vi "Calculate-value-shape.vi"(4 "Center index X":i32, 5 "Temperature field":dbl[][](array[numeric]), 6 "Center index Y":i32, 7 "Characteristics":T2[](array[typedef]), 8 "error in":errorcluster, 10 "Temp. params. ref. in":refnum<data-value>, 11 "Config. params. ref. in":refnum<data-value>) -> (0 "error IO":errorcluster, 1 "Temperature characteristics":T1 {"Stand. dev. temperature" format="%#.1f"; "Min. temperature" format="%#.0f"; "Max. temperature" format="%#.0f"; "Average temperature" format="%#.0f"}, 2 "Temp. params. ref. in":refnum<data-value>, 3 "Config. params. ref.":refnum<data-value>)   [LabVIEW 2013, in "CameraVision.lvlib" / "CV-Temperature.lvclass"]
uses:
  CV-Temperature.lvclass
  Analysis/Characteristics-cluster.ctl
  Configuration/CV-Configuration.lvclass
  Temperature-characteristics.ctl
  Configuration/CV-Configuration.lvclass/CV-Configuration.ctl
  CV-Temperature.lvclass/CV-Temperature.ctl
  <vilib>/Analysis/coordinate.llb/2D Cartesian Coordinate Shift (Scalar).vi
  <vilib>/Analysis/coordinate.llb/2D Cartesian Coordinate Rotation (Scalar).vi
  Read Averaging shape.vi
  Read Major axis.vi
  Read Minor axis.vi
  Configuration/Read ROI width.vi
  Configuration/Read ROI height.vi
  <vilib>/Analysis/NI_AALPro.lvlib
  Analysis/CV-Analysis.lvclass
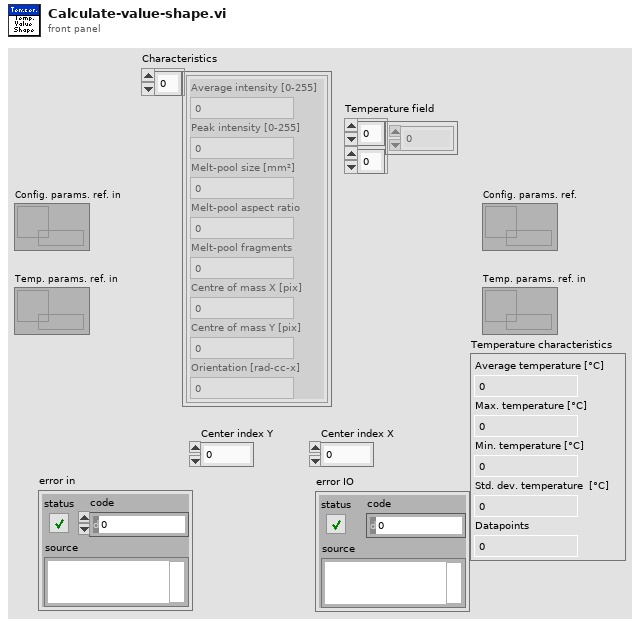
[diagram p1: front panel]
types:
  T1 = typedef "CameraVision.lvlib/CV-Temperature.lvclass/Temperature-characteristics.ctl" = cluster{"Average temperature ":dbl, "Max. temperature":dbl, "Min. temperature":dbl, "Stand. dev. temperature":dbl, "Datapoints":dbl}
  T2 = typedef "CameraVision.lvlib/CV-Analysis.lvclass/Characteristics-cluster.ctl" = cluster{"Average intensity":dbl, "Peak intensity":dbl, "Melt-pool size":dbl, "Melt-pool aspect ratio":dbl, "Melt-pool fragments":dbl, "Centre of mass X":dbl, "Centre of mass Y":dbl, "Orientation":dbl}
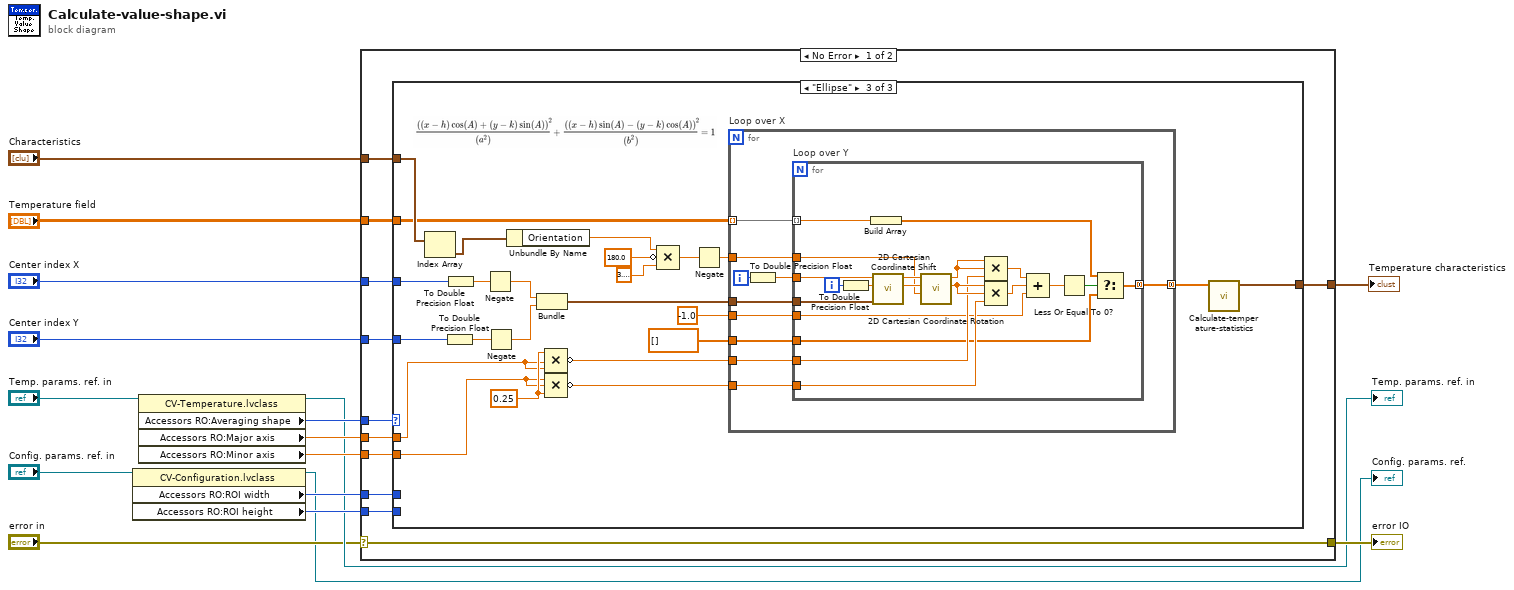
[diagram p0: block diagram]
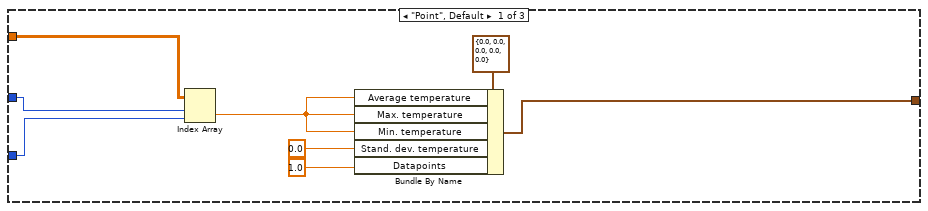
[diagram p2: hidden frame]
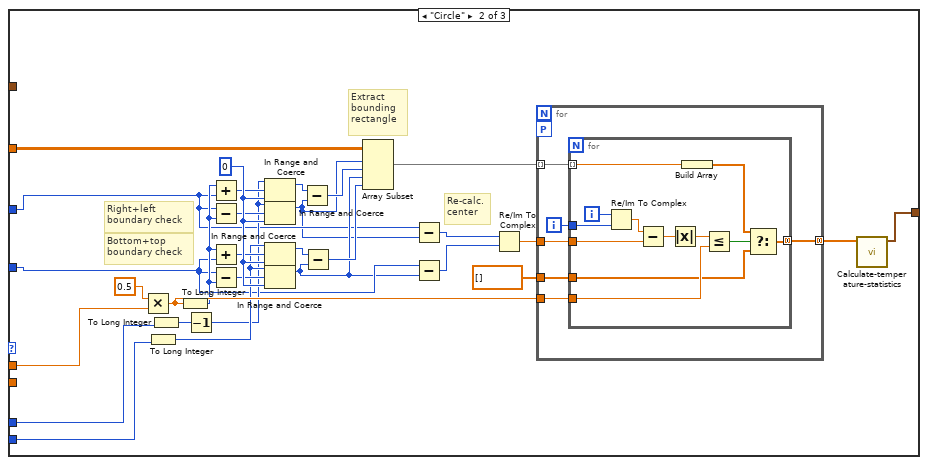
[diagram p3: hidden frame]
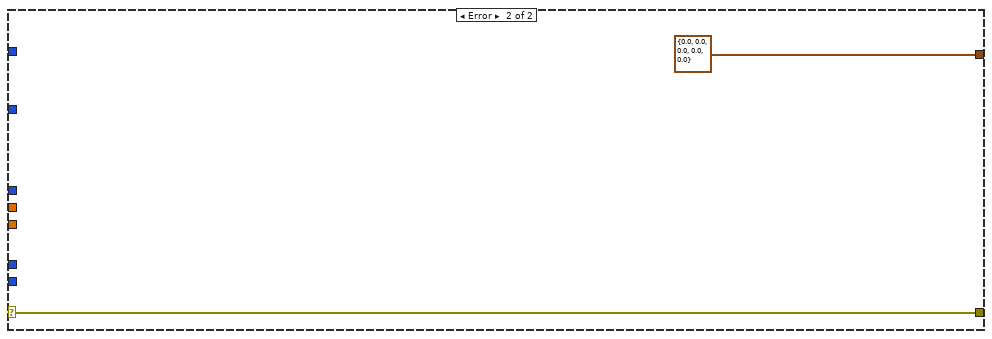
[diagram p4: hidden frame]
diagram:
  n1 = property class="CV-Configuration.lvclass"(reference="Config. params. ref. in") -> (reference out=→"Config. params. ref.":refnum<data-value>, "Accessors RO:ROI width"=w6:u32, "Accessors RO:ROI height"=w5:u32)  [unwired: 1 in, 1 out]
  n2 = property class="CV-Temperature.lvclass"(reference="Temp. params. ref. in") -> (reference out=→"Temp. params. ref. in":refnum<data-value>, "Accessors RO:Averaging shape"=w10:enum16{"Point", "Circle", "Ellipse"}, "Accessors RO:Major axis"=w9:dbl, "Accessors RO:Minor axis"=w8:dbl)  [unwired: 1 in, 1 out]
  n3 = case shown="No Error" "error in" {
    selector: "error in" -> [w23 w139]
    tunnel: [w27 T1 {"Average temperature "=0.0, "Max. temperature"=0.0, "Min. temperature"=0.0, "Stand. dev. temperature"=0.0, "Datapoints"=0.0} ("Temperature characteristics")] -> w2
    tunnel: "Center index Y" -> [w26 _]
    tunnel: "Center index X" -> [w25 _]
    tunnel: w10 -> [w24 _]
    tunnel: [w23 w139] -> w14
    tunnel: "Temperature field" -> [w22 _]
    tunnel: "Characteristics" -> [w21 _]
    tunnel: w9 -> [w20 _]
    tunnel: w8 -> [w19 _]
    tunnel: w6 -> [w18 _]
    tunnel: w5 -> [w17 _]
    frame No Error {
      n4 = case shown="\"Ellipse\"" w24 {
        tunnel: w25 -> [w35 w42 w106]
        tunnel: w26 -> [w34 w44 w105]
        tunnel: [w32 w62 w84] -> w27
        tunnel: w22 -> [w29 w40 w88]
        tunnel: w21 -> [_ _ w89]
        tunnel: w20 -> [_ w37 w87]
        tunnel: w19 -> [_ _ w86]
        tunnel: w18 -> [_ w39 _]
        tunnel: w17 -> [_ w38 _]
        frame "Point", Default {
          n5 = Index Array(array=w29, index (row)=w35, index (col)=w34) -> (element=w28:dbl)
          n6 = Bundle By Name(cluster=T1 {"Average temperature "=0.0, "Max. temperature"=0.0, "Min. temperature"=0.0, "Stand. dev. temperature"=0.0, "Datapoints"=0.0} ("Temperature characteristics"), "Average temperature"=w28, "Max. temperature"=w28, "Min. temperature"=w28, "Stand. dev. temperature"=0.0 ("Temperature characteristics.Stand. dev. temperature"), "Datapoints"=1.0 ("Temperature characteristics.Datapoints")) -> (w32:T1)
        }
        frame "Circle" {
          w57 = 0 ("lower limit")
          # "Re-calc.\ncenter"
          # "Extract \nbounding \nrectangle"
          # "Bottom+top \nboundary check"
          # "Right+left\nboundary check"
          n7 = Multiply(x=0.5, y=w37) -> (x*y=w61:dbl)
          n8 = To Long Integer(number=w38) -> (32bit integer=w49:i32)
          n9 = To Long Integer(number=w39) -> (32bit integer=w50:i32)
          n10 = To Long Integer(number=w61) -> (32bit integer=w47:i32)
          n11 = Decrement(x=w50) -> (x-1=w48:i32)
          n12 = Add(x=w47, y=w42) -> (x+y=w53:i32)
          n13 = Subtract(x=w42, y=w47) -> (x-y=w54:i32)
          n14 = Add(x=w47, y=w44) -> (x+y=w55:i32)
          n15 = Subtract(x=w44, y=w47) -> (x-y=w56:i32)
          n16 = In Range and Coerce(upper limit=w48, x=w53, lower limit=w57) -> (coerced(x)=w58:i32)  [unwired: 1 out]
          n17 = In Range and Coerce(upper limit=w48, x=w54, lower limit=w57) -> (coerced(x)=w41:i32)  [unwired: 1 out]
          n18 = In Range and Coerce(upper limit=w49, x=w55, lower limit=w57) -> (coerced(x)=w59:i32)  [unwired: 1 out]
          n19 = In Range and Coerce(upper limit=w49, x=w56, lower limit=w57) -> (coerced(x)=w43:i32)  [unwired: 1 out]
          n20 = Subtract(x=w58, y=w41) -> (x-y=w52:i32)
          n21 = Subtract(x=w59, y=w43) -> (x-y=w51:i32)
          n22 = Array Subset(array=w40, index (row)=w41, length (row)=w52, index (col)=w43, length (col)=w51) -> (w64:dbl[][])
          n23 = Subtract(x=w42, y=w41) -> (x-y=w46:i32)
          n24 = Subtract(x=w44, y=w43) -> (x-y=w45:i32)
          n25 = Re/Im To Complex(1:w45, 2:w46) -> (0:w63:cdb)
          n26 = for {
            tunnel: w64 -> [w71] mode=indexing
            tunnel: w63 -> [w69]
            tunnel: w61 -> [w68]
            tunnel: [w67] -> w36 mode=concatenating
            tunnel: dbl[] [] -> [w66]
            workers-P: _ -> [_]
            i -> [w70]
            n27 = for {
              tunnel: w71 -> [w72] mode=indexing
              tunnel: w70 -> [w82]
              tunnel: w69 -> [w80]
              tunnel: w68 -> [w78]
              tunnel: [w74] -> w67 mode=concatenating
              tunnel: w66 -> [w73]
              i -> [w83]
              n28 = Re/Im To Complex(1:w82, 2:w83) -> (0:w81:cdb)
              n29 = Subtract(x=w81, y=w80) -> (x-y=w79:cdb)
              n30 = Absolute Value(x=w79) -> (abs(x)=w77:dbl)
              n31 = Build Array(w72) -> (w75:dbl[])
              n32 = Less Or Equal?(x=w77, y=w78) -> (x <= y?=w76:bool)
              n33 = Select(t=w75, s=w76, f=w73) -> (s? t:f=w74:dbl[])
            }
          }
          n34 = call "Calculate-temperature-statistics.vi"("Temperature array"=w36) -> ("Temperature characteristics"=w62:T1)  [unwired: 10 in]
        }
        frame "Ellipse" {
          w104 = 0.25 ("x")
          n35 = Index Array(array=w89) -> (element=w107:T2)  [unwired: 1 in]
          n36 = To Double Precision Float(number=w105) -> (double precision float=w102:dbl)
          n37 = To Double Precision Float(number=w106) -> (double precision float=w103:dbl)
          n38 = Negate(x=w103) -> (-x=w101:dbl)
          n39 = Negate(x=w102) -> (-x=w100:dbl)
          n40 = Unbundle By Name(w107) -> ("Orientation"=w91:dbl)
          n41 = Bundle(w101, w100) -> (w99:cluster{dbl, dbl})  [unwired: 1 in]
          n42 = Compound Arithmetic op=MULTIPLY(w104, w87, w87) -> (invert w97:dbl)
          n43 = Compound Arithmetic op=MULTIPLY(w86, w86, w104) -> (invert w96:dbl)
          n44 = Compound Arithmetic op=MULTIPLY(w91, invert 180.0, 3.141592653589793) -> (w90:dbl)
          n45 = Negate(x=w90) -> (-x=w98:dbl)
          n46 = for "Loop over X" {
            tunnel: w88 -> [w117] mode=indexing
            tunnel: [w116] -> w85 mode=concatenating
            tunnel: w99 -> [w113]
            tunnel: w98 -> [w112]
            tunnel: w97 -> [w111]
            tunnel: w96 -> [w110]
            tunnel: -1.0 ("value") -> [w109]
            tunnel: dbl[] [] -> [w108]
            i -> [w115]
            n47 = To Double Precision Float(number=w115) -> (double precision float=w114:dbl)
            n48 = for "Loop over Y" {
              tunnel: w117 -> [w118] mode=indexing
              tunnel: [w121] -> w116 mode=concatenating
              tunnel: w114 -> [w137]
              tunnel: w113 -> [w134]
              tunnel: w112 -> [w126]
              tunnel: w111 -> [w125]
              tunnel: w110 -> [w124]
              tunnel: w109 -> [w120]
              tunnel: w108 -> [w119]
              i -> [w136]
              n49 = To Double Precision Float(number=w136) -> (double precision float=w135:dbl)
              n50 = Build Array(w118) -> (w122:dbl[])
              n51 = call-poly <vilib>:"2D Cartesian Coordinate Shift.vi"("shift"=w134, "y"=w135, "x"=w137) -> ("y out"=w127:dbl, "x out"=w128:dbl)  [unwired: 6 in, 1 out]
              n52 = call-poly <vilib>:"2D Cartesian Coordinate Rotation.vi"("theta"=w126, "y"=w127, "x"=w128) -> ("y out"=w129:dbl, "x out"=w130:dbl)  [unwired: 6 in, 1 out]
              n53 = Compound Arithmetic op=MULTIPLY(w130, w130, w125) -> (w133:dbl)
              n54 = Compound Arithmetic op=MULTIPLY(w129, w129, w124) -> (w132:dbl)
              n55 = Compound Arithmetic op=ADD(w133, w132, w120) -> (w131:dbl)
              n56 = Less Or Equal To 0?(x=w131) -> (x <= 0?=w123:bool)
              n57 = Select(t=w122, s=w123, f=w119) -> (s? t:f=w121:dbl[])
            }
          }
          n58 = call "Calculate-temperature-statistics.vi"("Temperature array"=w85) -> ("Temperature characteristics"=w84:T1)  [unwired: 10 in]
        }
      }
    }
    frame Error {
    }
  }
  "error IO" <- w14
  "Temperature characteristics" <- w2
